vi "event data analysis start.vi"(0 "position in [km]":sgl, 11 "times in":T3[](array[typedef])) -> (2 "average event":T1={"position [km]"=1077.0, "time [nsec]"=105087035626983}, 4 "events":T1[](array[typedef]), 8 "num of events":i32=12, 13 "histogram":T2(graph), 14 "standard deviation (ns)":i32=7678, 15 "mean time (ns)":dbl=105087000000000.0)   [LabVIEW 2014]
doc: "event data analysis start (BAE4)\n\nTakes time and position as input and returns average, mean, and standard deviation of times, along with bundled data of events, a histogram, and the amount of input data.\n\nBeverly Abadines\nPHY 350\nE4"
uses:
  typedefs/time cluster typedef.ctl
  typedefs/event cluster typedef.ctl
  <vilib>/Analysis/NI_AALBase.lvlib
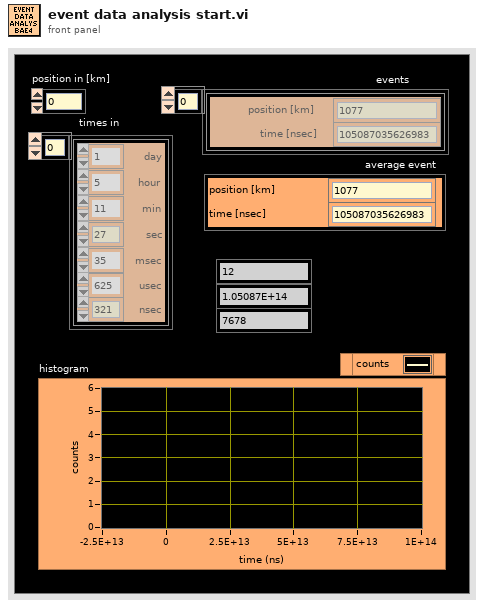
[diagram p1: front panel]
types:
  T1 = typedef "event cluster typedef.ctl" = cluster{"position [km]":sgl, "time [nsec]":i64}
  T2 = cluster{"X Values":dbl[], "Histogram: h(x)":i32[]}
  T3 = typedef "time cluster typedef.ctl" = cluster{"day":u32, "hour":u32, "min":u32, "sec":u32, "msec":u32, "usec":u32, "nsec":u32}
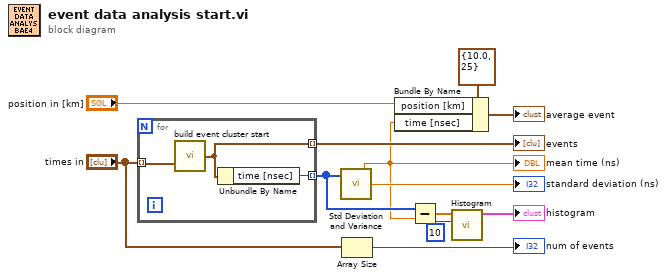
[diagram p0: block diagram]
diagram:
  n1 = for {
    tunnel: "times in" -> [w15] mode=indexing
    tunnel: [w14] -> w9 mode=indexing
    tunnel: [w13] -> w5 mode=indexing
    n2 = call "build event cluster start.vi"("time cluster in"=w15) -> ("event data out"=w13:T1)  [unwired: 14 in]
    n3 = Unbundle By Name(w13) -> ("time [nsec]"=w14:i64)
  }
  "events" <- w5
  n4 = call <vilib>:"Std Deviation and Variance.vi"("X"=w9) -> ("mean"=w1:dbl, "standard deviation"=→"standard deviation (ns)":dbl)  [unwired: 1 in, 1 out]
  "mean time (ns)" <- w1
  n5 = Array Size(array="times in") -> (size(s)=→"num of events":i32)
  n6 = Bundle By Name(cluster=T1 {"position [km]"=10.0, "time [nsec]"=25} ("average event"), "position [km]"="position in [km]", "time [nsec]"=w1) -> (→"average event":T1)
  n7 = Subtract(x=w9, y=w1) -> (x-y=w7:dbl[])
  n8 = call <vilib>:"Histogram.vi"("intervals"=10 ("y"), "X"=w7) -> ("Histogram Graph"=→"histogram":T2)  [unwired: 6 in, 3 out]
